vi "Event Next Frame.vi"(0 "Diagram in":refnum<vi>, 5 "Event Data Out Names":string[](array[string]), 7 "Event Data out":refnum<vi>[](array[refnum]), 9 "Event Data In Names":string[](array[string]), 11 "error in (no error)":errorcluster) -> (4 "Selected Diagram":refnum<vi>, 6 "Inputs":refnum<vi>[](array[refnum]), 8 "Event Data in":refnum<vi>[](array[refnum]), 15 "error out":errorcluster)   [LabVIEW 2015, in "Scripting.lvlib"]
doc: "Navigates to the next frame of the Event Structure that owns <B>Diagram in</B>, supplying the frame's diagram at <B>Diagram out</B>.\n\n<B>Event Data Out Names</B> are the names of the desired Event Data out elements of the current frame.\n\n<B>Event Data Out<B> is an array of terminals to wire to the configured Event Data out terminals.\n\n<B>Event Data in Names</B> are the names of the desired Event Data in elements of the next frame.\n\n<B>Event Data in</B> is an array containing the configured terminals of the Event Data in node of the next frame."
uses:
  Scripting.lvlib
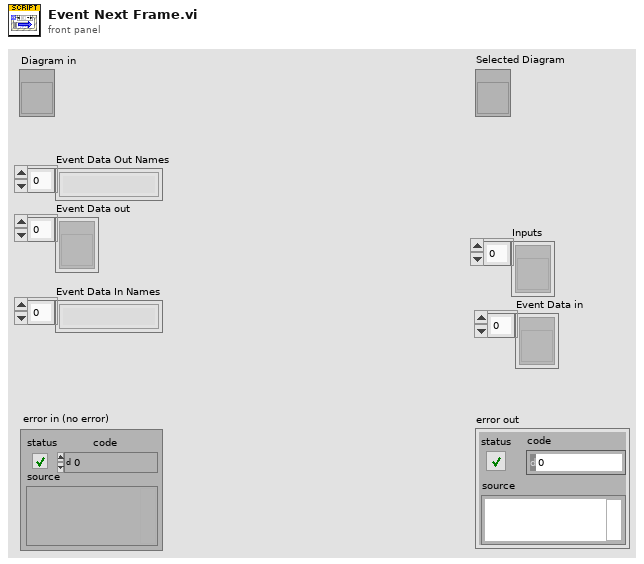
[diagram p1: front panel]
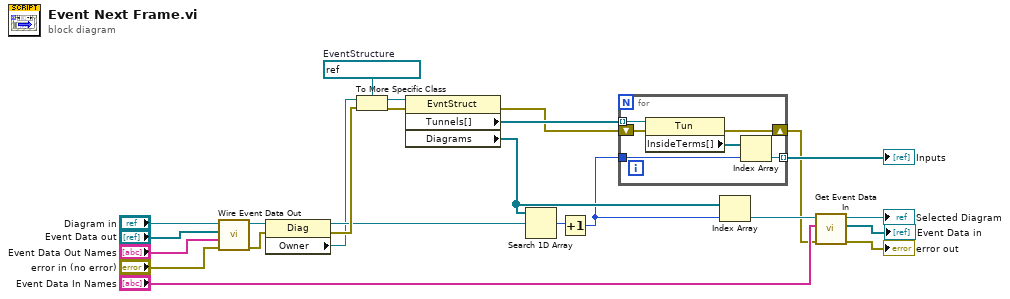
[diagram p0: block diagram]
diagram:
  w23 = refnum<vi> refnum  # EventStructure
  n1 = call "Wire Event Data Out.vi"("error in (no error)"="error in (no error)", "Event Data Names"="Event Data Out Names", "Event Data"="Event Data out", "Diagram in"="Diagram in") -> ("error out"=w10:errorcluster, "Diagram out"=w8:refnum<vi>)  [unwired: 6 in]
  n2 = property class="Diag"(reference=w8, error in=w10) -> (reference out=w7:refnum<vi>, error out=w9:errorcluster, "Owner"=w6:refnum<vi>)
  n3 = To More Specific Class(target class=w23, reference=w6, error in=w9) -> (specific class reference=w14:refnum<vi>, error out=w13:errorcluster)
  n4 = property class="EvntStruct"(reference=w14, error in=w13) -> (error out=w15:errorcluster, "Tunnels[]"=w16:refnum<vi>[], "Diagrams"=w19:refnum<vi>[])  [unwired: 1 out]
  n5 = Search 1D Array(1D array=w19, element=w7) -> (index of element=w18:i32)  [unwired: 1 in]
  n6 = Increment(x=w18) -> (x+1=w17:i32)
  n7 = for {
    tunnel: w16 -> [w30] mode=indexing
    tunnel: w17 -> [w28]
    shift-right: [w26] -> w3
    shift-left: w15 -> [w27]
    tunnel: [w25] -> w22 mode=indexing
    n8 = property class="Tun"(reference=w30, error in=w27) -> (error out=w26:errorcluster, "InsideTerms[]"=w29:refnum<vi>[])  [unwired: 1 out]
    n9 = Index Array(array=w29, index=w28) -> (element=w25:refnum<vi>)
  }
  "Inputs" <- w22
  n10 = Index Array(array=w19, index=w17) -> (element=w24:refnum<vi>)
  n11 = call "Get Event Data In.vi"("error in (no error)"=w3, "Event Data Names"="Event Data In Names", "Diagram in"=w24) -> ("error out"=→"error out":errorcluster, "OutputTerms[]"=→"Event Data in":refnum<vi>[], "Diagram out"=→"Selected Diagram":refnum<vi>)  [unwired: 6 in]
